vi "Get_MSI.vi"(8 "error in (no error)":errorcluster, 11 "IB_MSI in":refnum<class "IB_MSI.lvclass">) -> (0 "error out":errorcluster, 2 "data":T1={"upgradeCode"="", "distID"="", "windowMessage"="", "windowTitle"="", "arpPhone"="", "arpContact"="", "arpURL"="http://", "arpCompany"="", "licenseID"="", "licensePath"=path "", "welcomeImageID"="", "welcomeImagePath"=path "", "bannerImageID"="", "bannerImagePath"=path "", "osCheck"=0, "msiFileName"="", "cabFileName"="", "hwOption"=enum."<none>", "hwPath"=path "", "regGroup"=[], "regDest"=[], "selectedDists"=[], "installedDists"=[], "postInstallSteps"=[], "preUninstallSteps"=[], "winsec.certificate"="", "winsec.timestamp"="", "winsec.description"="", "autoselect drivers"=FALSE, "hide non-runtimes"=FALSE}, 3 "IB_MSI out":refnum<class "IB_MSI.lvclass">)   [LabVIEW 2020, in "IB_MSI.lvclass"]
uses:
  <vilib>/AppBuilder/IB_Classes/MSI/IB_MSI.lvclass
  <vilib>/AppBuilder/IB_Classes/MSI/IB_MSI.lvclass/IB_MSI.ctl
  <resource>/Framework/Providers/Builds/Installer/CDK_sTypeDef_HWImportOption.ctl
  <vilib>/AppBuilder/IB_Classes/RegDest/IB_RegDest.lvclass
  <vilib>/AppBuilder/IB_Classes/DistPart/IB_DistPart.lvclass
  <vilib>/AppBuilder/IB_Classes/MSI/IB_MSI.ctl
  <vilib>/AppBuilder/IB_Classes/RegGroup/IB_RegGroup.lvclass
  <vilib>/AppBuilder/IB_Classes/Post_Install_Step/IB_Post_Install_Step.lvclass
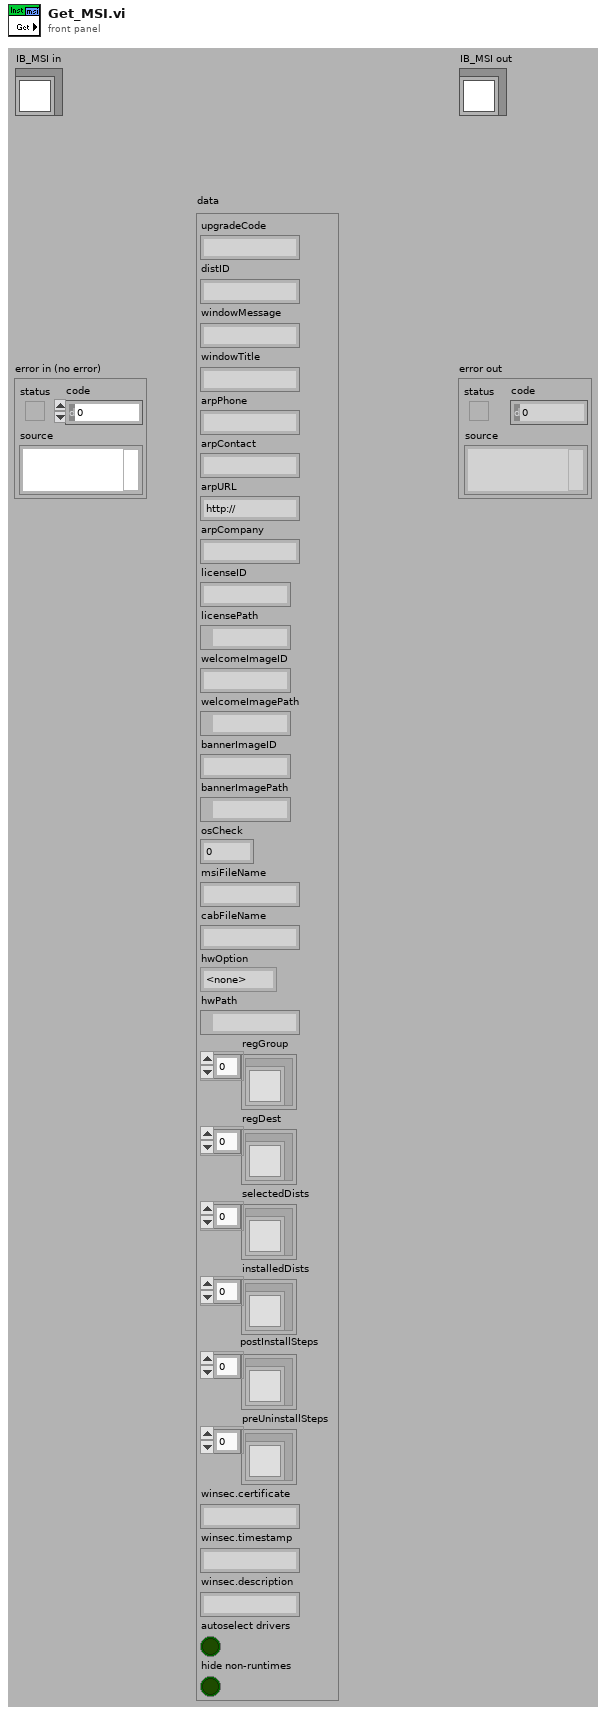
[diagram p1: front panel]
types:
  T1 = typedef "IB_MSI.ctl" = cluster{"upgradeCode":string, "distID":string, "windowMessage":string, "windowTitle":string, "arpPhone":string, "arpContact":string, "arpURL":string, "arpCompany":string, "licenseID":string, "licensePath":path, "welcomeImageID":string, "welcomeImagePath":path, "bannerImageID":string, "bannerImagePath":path, "osCheck":i32, "msiFileName":string, "cabFileName":string, "hwOption":T2, "hwPath":path, "regGroup":refnum<class "IB_RegGroup.lvclass">[], "regDest":refnum<class "IB_RegDest.lvclass">[], "selectedDists":refnum<class "IB_DistPart.lvclass">[], "installedDists":refnum<class "IB_DistPart.lvclass">[], "postInstallSteps":refnum<class "IB_Post_Install_Step.lvclass">[], "preUninstallSteps":refnum<class "IB_Post_Install_Step.lvclass">[], "winsec.certificate":string, "winsec.timestamp":string, "winsec.description":string, "autoselect drivers":bool, "hide non-runtimes":bool}
  T2 = typedef "CDK_sTypeDef_HWImportOption.ctl" = enum16{"<none>", "Merge", "Replace", "Dialog"}
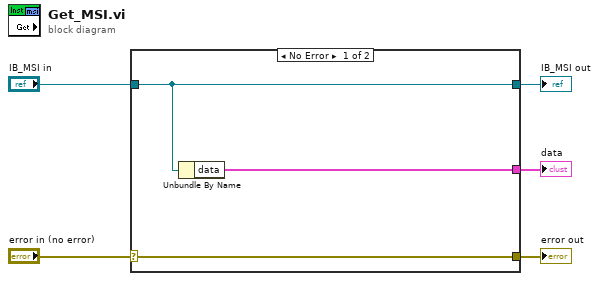
[diagram p0: block diagram]
diagram:
  n1 = case shown="No Error" "error in (no error)" {
    selector: "error in (no error)" -> [w8 w9]
    tunnel: [w8 w9] -> w4
    tunnel: [w7 w10] -> w2
    tunnel: "IB_MSI in" -> [w7 w10]
    tunnel: [w6 _] -> w1
    frame No Error {
      n2 = Unbundle By Name(w7) -> ("data"=w6:T1)
    }
    frame Error {
    }
  }
  "error out" <- w4
  "IB_MSI out" <- w2
  "data" <- w1
